vi "WorkorderHandler_QueueToObjectReference.vi"(1 "queue":refnum<queue>) -> (21 "reference":T1)   [LabVIEW 2011]
doc: "Converts a queue object refnum to a dqGOOP refnum"
uses:
  DataStructures/WorkorderHandler_ObjectData.ctl
  DataStructures/WorkorderHandler_ObjectReference.ctl
panel:
  in  "reference (default)":T1
  # "Copyright (C) 2004 DataAct Incorporated"
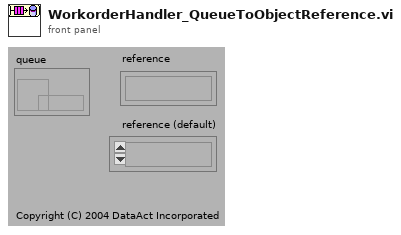
[diagram p1: front panel]
types:
  T1 = typedef "WorkorderHandler_ObjectReference.ctl" = refnum<k1>
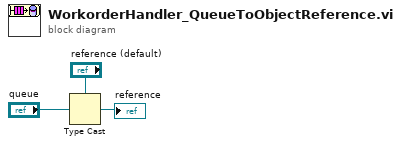
[diagram p0: block diagram]
diagram:
  n1 = Type Cast(type="reference (default)", x="queue") -> (*(type *) &x=→"reference":T1)
